vi "ContinueTorF(SubVI).vi"(10 "AdminNo":string) -> (3 "Boolean":bool)   [LabVIEW 2013]
uses:
  <vilib>/addons/database/Connection.llb/DB Tools Open Connec (String).vi
  <vilib>/addons/database/_DB Variant To Data/Database Variant To Data.xnode
  <vilib>/addons/database/NI_Database_API.lvlib
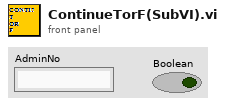
[diagram p1: front panel]
types:
  T1 = typedef "NI_Database_API.lvlib/Conn ObjectReference.ctl" = refnum<k1>
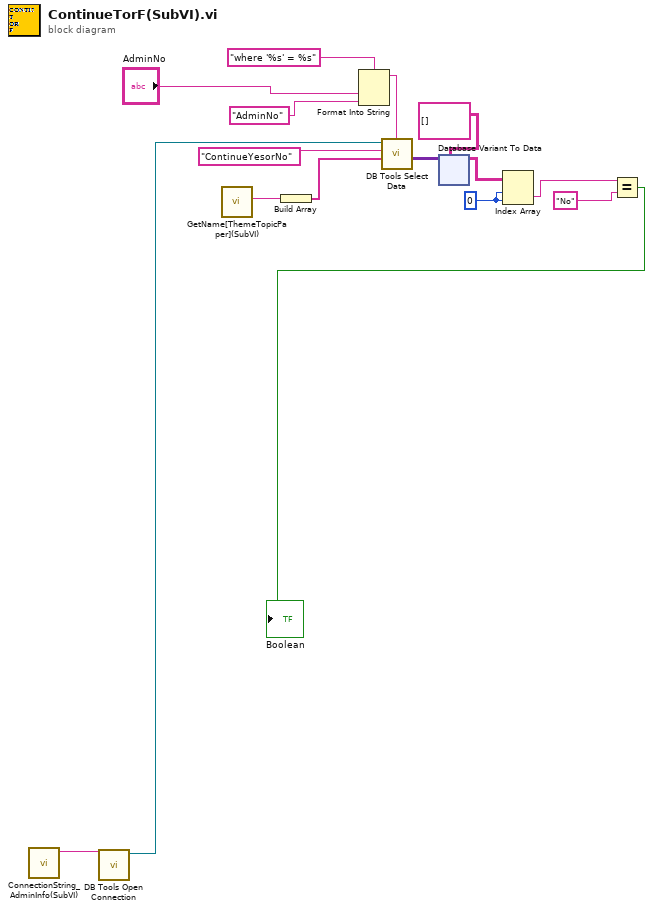
[diagram p0: block diagram]
diagram:
  w12 = 0 ("disabled index (col)")
  n1 = call "ConnectionString_AdminInfo(SubVI).vi"() -> ("ConnectionString"=w2:string)  [unwired: 11 in]
  n2 = call-poly <vilib>:"DB Tools Open Connection.vi"("connection information"=w2) -> ("connection reference"=w1:T1)  [unwired: 7 in, 1 out]
  n3 = call "GetName[ThemeTopicPaper](SubVI).vi"() -> ("Path for Score Table"=w4:string)  [unwired: 11 in]
  n4 = Build Array(w4) -> (w5:string[])
  n5 = Format Into String(format string="where '%s' = %s", "AdminNo", "AdminNo") -> (resulting string=w8:string)  [unwired: 2 in, 1 out]
  n6 = call <vilib>:"DB Tools Select Data.vi"("condition"=w8, "columns"=w5, "table"="ContinueYesorNo", "connection reference"=w1) -> ("data"=w13:variant[][])  [unwired: 2 in, 2 out]
  n7 = xnode "Database Variant To Data"("database variant"=w13, "type"=string[][] []) -> ("data"=w11:string[][])  [unwired: 1 in, 1 out]
  n8 = Index Array(array=w11, index (row)=w12, index (col)=w12) -> (element=w14:string)
  n9 = Equal?(x=w14, y="No") -> (x = y?=→"Boolean":bool)
